vi "Implement.vi"(0 "reference in":refnum<class "G#MethodTemplates.lvclass">, 5 "error in (no error)":errorcluster) -> (14 "reference out":refnum<class "G#MethodTemplates.lvclass">, 19 "error out":errorcluster)   [LabVIEW 2020, in "G#MethodTemplates.lvclass"]
uses:
  G#MethodTemplates.lvclass
  G#Interface/G#Interface.lvclass
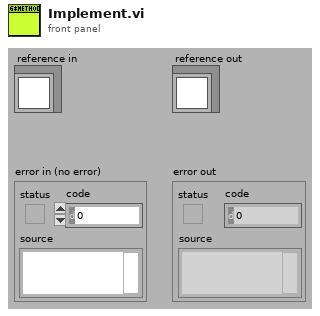
[diagram p1: front panel]
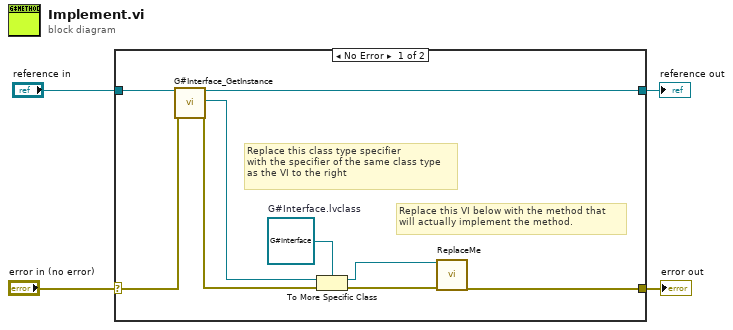
[diagram p0: block diagram]
diagram:
  n1 = case shown="No Error" "error in (no error)" {
    selector: "error in (no error)" -> [w11 w15]
    tunnel: [w7 w15] -> w3
    tunnel: [w12 w14] -> w1
    tunnel: "reference in" -> [w13 w14]
    frame No Error {
      w6 = refnum<class "G#Interface.lvclass"> refnum  # G#Interface.lvclass
      # "Replace this class type specifier\nwith the specifier of the same class type\nas the VI to the right"
      # "Replace this VI below with the method that\nwill actually implement the method."
      n2 = call-dynamic "G#Interface_GetInstance.vi"("reference in"=w13, "error in (no error)"=w11) -> ("reference out"=w12:refnum<class "G#MethodTemplates.lvclass">, "G#Object"=w9:refnum<class "G#Object.lvclass">, "error out"=w10:errorcluster)  [unwired: 14 in, 1 out]
      n3 = To More Specific Class(target class=w6, reference=w9, error in=w10) -> (specific class reference=w5:refnum<class "G#Interface.lvclass">, error out=w8:errorcluster)
      n4 = call "ReplaceMe.vi"("reference in"=w5, "error in (no error)"=w8) -> ("error out"=w7:errorcluster)  [unwired: 16 in, 1 out]
    }
    frame Error {
    }
  }
  "error out" <- w3
  "reference out" <- w1
